vi "lvlibp_FD_MatchPatterns.vi"(10 "patterns":string="*", 11 "qualified name":string) -> (3 "match?":bool)   [LabVIEW 2016]
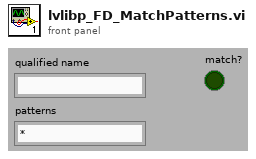
[diagram p1: front panel]
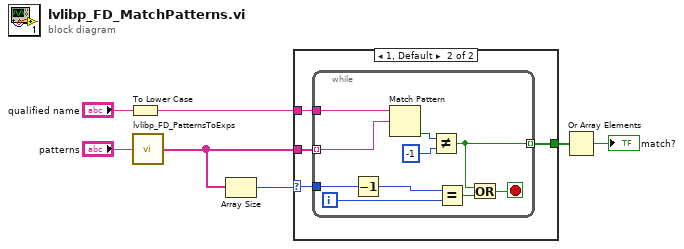
[diagram p0: block diagram]
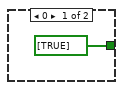
[diagram p2: hidden frame]
diagram:
  n1 = To Lower Case(string="qualified name") -> (all lower case string=w1:string)
  n2 = call <resource>:"lvlibp_FD_PatternsToExps.vi"("patterns"="patterns") -> ("array of regular expressions"=w4:string[])
  n3 = Array Size(array=w4) -> (size(s)=w3:i32)
  n4 = case shown="1, Default" w3 {
    selector: w3 -> [_ w10]
    tunnel: w4 -> [_ w12]
    tunnel: [bool[] [TRUE] w11] -> w6
    tunnel: w1 -> [_ w9]
    frame 0 {
    }
    frame 1, Default {
      n5 = while {
        tunnel: w12 -> [w22] mode=indexing
        tunnel: [w19] -> w11 mode=indexing
        tunnel: w10 -> [w15]
        tunnel: w9 -> [w13]
        i -> [w17]
        stop <- w16 stop-if-true
        n6 = Decrement(x=w15) -> (x-1=w14:i32)
        n7 = Match Pattern(string=w13, regular expression=w22) -> (offset past match=w21:i32)  [unwired: 1 in, 3 out]
        n8 = Not Equal?(x=w21, y=-1) -> (x != y?=w19:bool)
        n9 = Equal?(x=w14, y=w17) -> (x = y?=w18:bool)
        n10 = Or(x=w19, y=w18) -> (x .or. y?=w16:bool)
      }
    }
  }
  n11 = Or Array Elements(Boolean array=w6) -> (logical OR=→"match?":bool)
